vi "Is New Command.vi"(8 "error in (no error)":errorcluster, 11 "System in":refnum<class "System.lvclass">) -> (0 "error out":errorcluster, 2 "New Command":bool, 3 "System out":refnum<class "System.lvclass">)   [LabVIEW 2013, in "System.lvclass"]
uses:
  System.lvclass
  System.lvclass/System.ctl
  Commands/Command/Command.lvclass
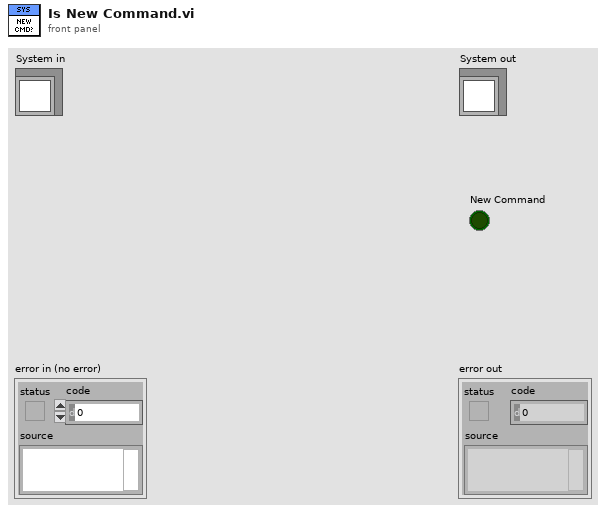
[diagram p1: front panel]
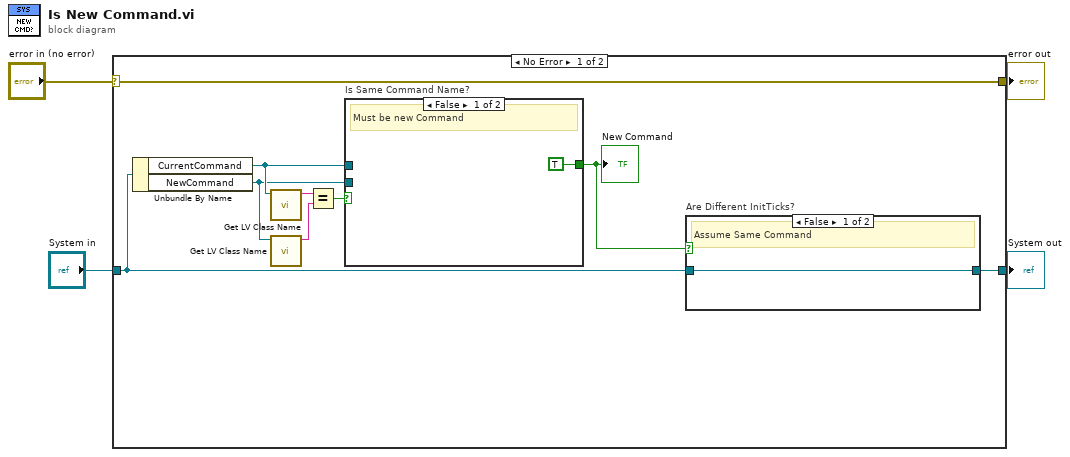
[diagram p0: block diagram]
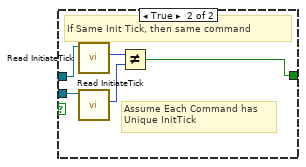
[diagram p2: hidden frame]
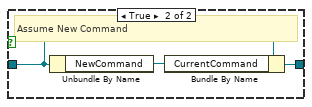
[diagram p3: hidden frame]
diagram:
  n1 = case shown="No Error" "error in (no error)" {
    selector: "error in (no error)" -> [w11 w25]
    tunnel: [w11 w25] -> w3
    tunnel: [w12 w24] -> w1
    tunnel: "System in" -> [w13 w24]
    frame No Error {
      n2 = Unbundle By Name(w13) -> ("CurrentCommand"=w7:refnum<class "Command.lvclass">, "NewCommand"=w6:refnum<class "Command.lvclass">)
      n3 = call <vilib>:"Get LV Class Name.vi"("object"=w7) -> ("class name"=w10:string)  [unwired: 9 in, 1 out]
      n4 = call <vilib>:"Get LV Class Name.vi"("object"=w6) -> ("class name"=w9:string)  [unwired: 9 in, 1 out]
      n5 = Equal?(x=w10, y=w9) -> (x = y?=w8:bool)
      n6 = case "Is Same Command Name?" shown="False" w8 {
        tunnel: w7 -> [_ w17]
        tunnel: w6 -> [_ w16]
        tunnel: [TRUE w15] -> w5
        frame False {
          # "Must be new Command"
        }
        frame True {
          # "Assume Each Command has\nUnique InitTick"
          # "If Same Init Tick, then same command"
          n7 = call-dynamic "Read InitiateTick.vi"("Command in"=w17) -> ("InitiateTick"=w19:u32)  [unwired: 8 in, 2 out]
          n8 = call-dynamic "Read InitiateTick.vi"("Command in"=w16) -> ("InitiateTick"=w18:u32)  [unwired: 8 in, 2 out]
          n9 = Not Equal?(x=w19, y=w18) -> (x != y?=w15:bool)
        }
      }
      "New Command" <- w5
      n10 = case "Are Different InitTicks?" shown="False" w5 {
        tunnel: w13 -> [w20 w23]
        tunnel: [w20 w22] -> w12
        frame False {
          # "Assume Same Command"
        }
        frame True {
          # "Assume New Command"
          n11 = Unbundle By Name(w23) -> ("NewCommand"=w21:refnum<class "Command.lvclass">)
          n12 = Bundle By Name(cluster=w23, "CurrentCommand"=w21) -> (w22:refnum<class "System.lvclass">)
        }
      }
    }
    frame Error {
    }
  }
  "error out" <- w3
  "System out" <- w1
